vi "Init Msg.vi"(10 "Msg Input":refnum<class "Msg Input.lvclass">) -> (2 "Msg":refnum<class "Msg.lvclass">)   [LabVIEW 2025, in "jettl.lvlib" / "Stopped jettl Msg.lvlib" / "Stopped Msg.lvlib"]
uses:
  Stopped Msg.lvlib
  Stopped Msg/Stopped Msg.lvclass
  Msg/Msg.lvclass
  Msg Input/Msg Input.lvclass
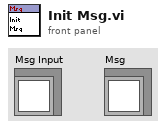
[diagram p1: front panel]
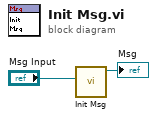
[diagram p0: block diagram]
diagram:
  n1 = call "Init Msg.vi"("Msg Input"="Msg Input") -> ("Stopped Msg out"=→"Msg":refnum<class "Stopped Msg.lvclass">)  [unwired: 10 in]
